vi "st_str Set Visable on Multiple Controls.vi"(10 "Visable?":bool, 11 "Controls":refnum<vi>[](array[refnum])) -> ()   [LabVIEW 2017]
doc: "Sets all the controls in the input array to the \"Enable state\" value."
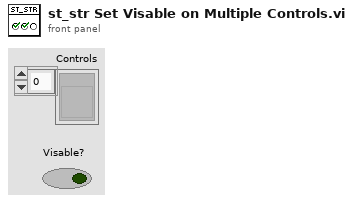
[diagram p1: front panel]
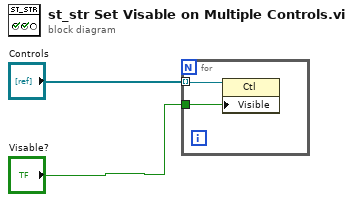
[diagram p0: block diagram]
diagram:
  n1 = for {
    tunnel: "Controls" -> [w4] mode=indexing
    tunnel: "Visable?" -> [w3]
    n2 = property class="Ctl"(reference=w4, "Visible"=w3) -> ()  [unwired: 1 in, 2 out]
  }
